vi "generate_sin_point.vi"(1 "Point Index":i32, 2 "Fout":dbl=1000000.0, 3 "Offset":dbl, 4 "Phase":dbl, 5 "Amp":dbl=2.0, 6 "Freq":dbl=500.0) -> (0 "Point Value":dbl)   [LabVIEW 2010]
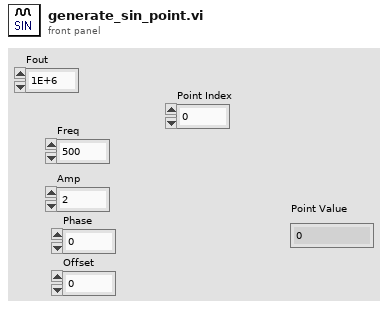
[diagram p1: front panel]
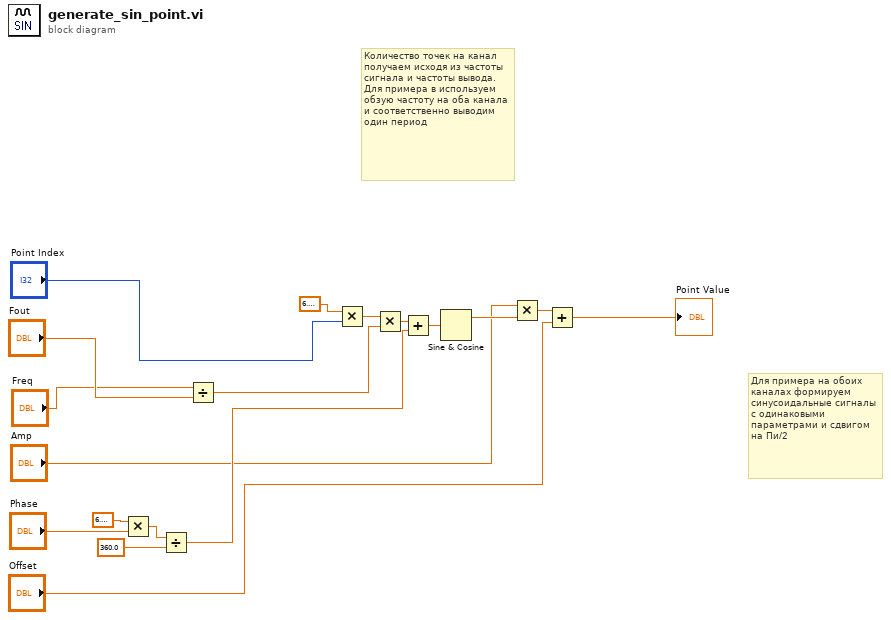
[diagram p0: block diagram]
diagram:
  # "Для примера на обоих каналах формируем синусоидальные сигналы с одинаковыми параметрами и сдвигом на Пи/2"
  # "Количество точек на канал получаем исходя из частоты сигнала и частоты вывода. Для примера в используем обзую частоту на оба канала и соответственно выводим один период"
  n1 = Multiply(x=6.283185307179586, y="Phase") -> (x*y=w16:dbl)
  n2 = Divide(x=w16, y=360.0) -> (x/y=w4:dbl)
  n3 = Divide(x="Freq", y="Fout") -> (x/y=w7:dbl)
  n4 = Multiply(x=6.283185307179586, y="Point Index") -> (x*y=w6:dbl)
  n5 = Multiply(x=w6, y=w7) -> (x*y=w5:dbl)
  n6 = Add(x=w5, y=w4) -> (x+y=w10:dbl)
  n7 = Sine & Cosine(0:w10) -> (1:w11:dbl)  [unwired: 1 out]
  n8 = Multiply(x="Amp", y=w11) -> (x*y=w9:dbl)
  n9 = Add(x=w9, y="Offset") -> (x+y=→"Point Value":dbl)
